vi "version_write.vi"(8 "error in (no error)":errorcluster, 10 "version":string, 11 "lv-build in":refnum<class "lv-builder.lvclass">) -> (0 "error out":errorcluster, 3 "lv-build out":refnum<class "lv-builder.lvclass">)   [LabVIEW 2015, in "lv-builder.lvclass"]
uses:
  lv-builder.lvclass
  lv-builder.lvclass/lv-builder.ctl
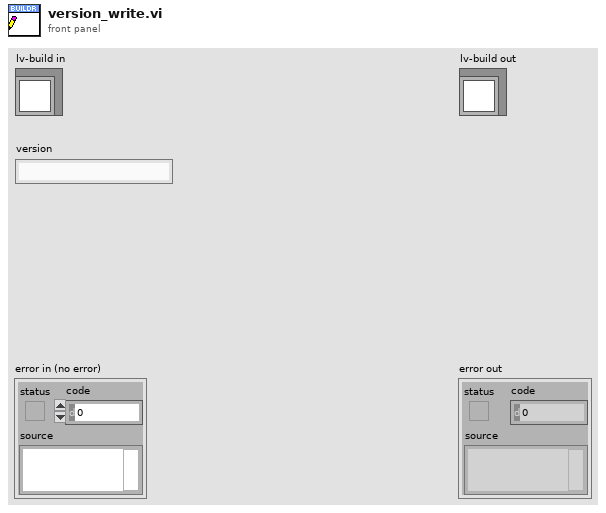
[diagram p1: front panel]
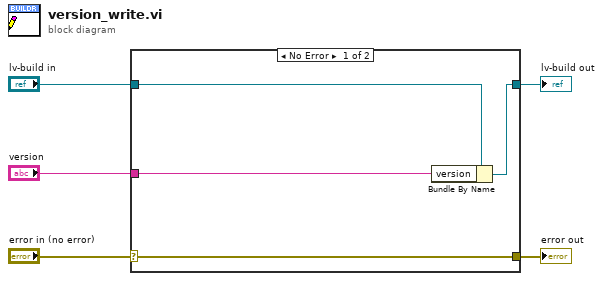
[diagram p0: block diagram]
diagram:
  n1 = case shown="No Error" "error in (no error)" {
    selector: "error in (no error)" -> [w9 w10]
    tunnel: [w9 w10] -> w4
    tunnel: [w7 w11] -> w2
    tunnel: "lv-build in" -> [w8 w11]
    tunnel: "version" -> [w6 _]
    frame No Error {
      n2 = Bundle By Name(cluster=w8, "version"=w6) -> (w7:refnum<class "lv-builder.lvclass">)
    }
    frame Error {
    }
  }
  "error out" <- w4
  "lv-build out" <- w2
